vi "Thread@ForeachBreak__Parameter.vi"(1 "ParamterIn":string) -> (0 "ParamterOut":string)   [LabVIEW 2019]
panel:
  out "Variable List":string[](array[string])
  in  "Confirm":bool
  out "IO List":string[](array[string])
  in  "IOLogic":string(combo)
  # "Thread@ForeachBreak $IOLogic\nIOLogic Express is:\nIO1 & (IO2 | IO3)\nVar==XXX, !=XXX, >=XXX, <=XXX, >XXX, <XXX\nVar <> XXX~YYY, </>XXX~YYY\nVar==NULL, ==EXIST, ==[],==[;;]\n~IOLogic will inverse Logic"
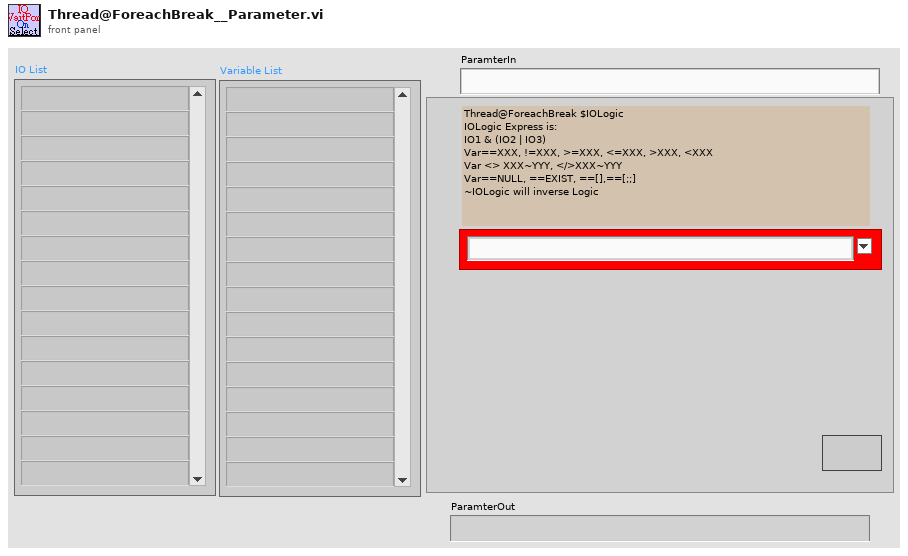
[diagram p1: front panel]
types:
  T1 = enum16{"Get", "Init", "Set", "Delete", "GetElement", "Inc", "Dec", "ReName"}
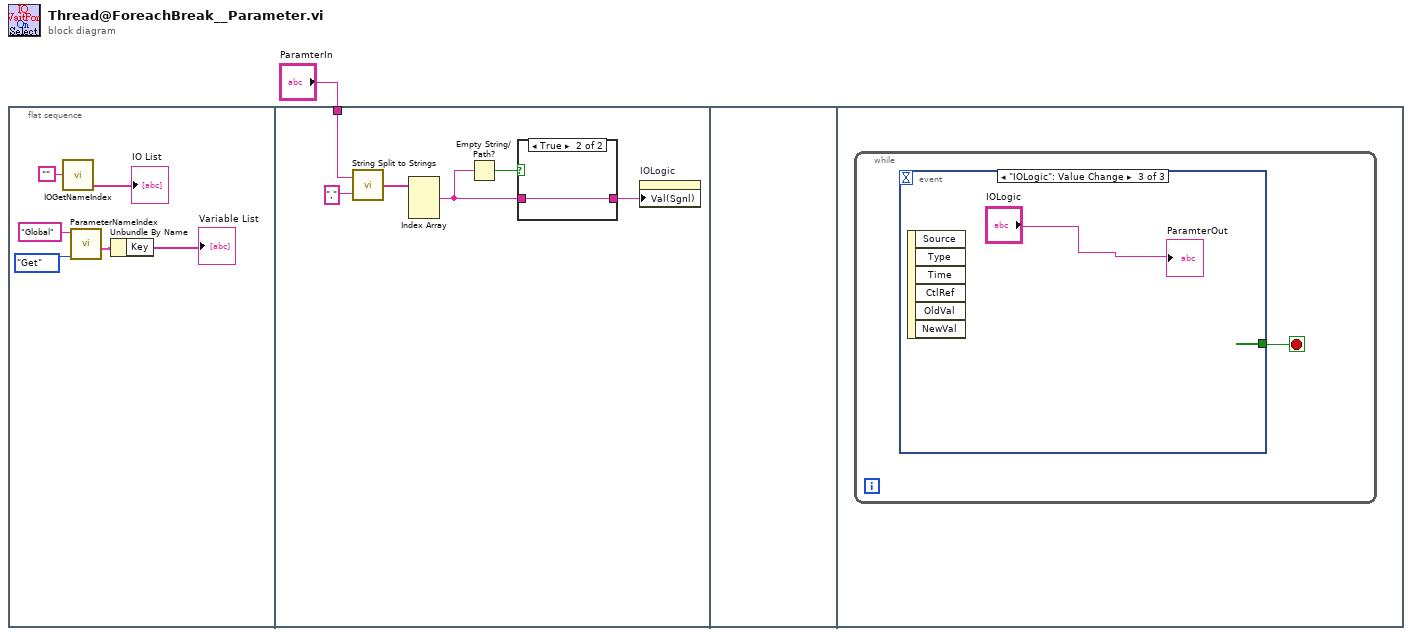
[diagram p0: block diagram]
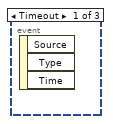
[diagram p3: hidden frame]
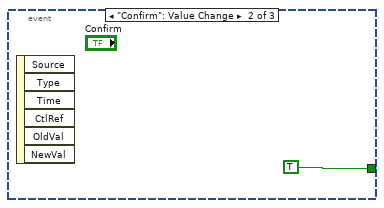
[diagram p4: hidden frame]
diagram:
  n1 = flat-sequence {
    tunnel: "ParamterIn" -> [w12]
    frame #0 {
      n2 = call "IOGetNameIndex.vi"("PortName"="") -> ("PortNameList Out"=→"IO List":string[])  [unwired: 3 in, 1 out]
      n3 = call "ParameterNameIndex.vi"("OP"=T1."Get", "VariableSection"="Global") -> ("GlobalKeyValue"=w4:cluster{"Key":string[], "Value":string[]})  [unwired: 3 in, 6 out]
      n4 = Unbundle By Name(w4) -> ("Key"=→"Variable List":string[])
    }
    frame #1 {
      n5 = call "String Split to Strings.vi"("search string/char (-)"=",", "String"=w12) -> ("Array"=w11:string[])
      n6 = Index Array(array=w11) -> (element #1=w9:string)  [unwired: 3 in, 2 out]
      n7 = Empty String/Path?(string/path=w9) -> (empty?=w10:bool)
      n8 = case shown="True" w10 {
        tunnel: w9 -> [w14 w15]
        tunnel: [w14 w15] -> w8
        frame False {
        }
        frame True {
        }
      }
      n9 = property on="IOLogic" class="CmbBox"("Val(Sgnl)"=w8) -> ()  [unwired: 2 in, 2 out]
    }
    frame #2 {
    }
    frame #3 {
      n10 = while {
        stop <- w16 stop-if-true
        n11 = event shown="[2] \"IOLogic\": Value Change" {
          selector: _ -> [_ _ _]
          dyn-events: _ -> [_ _ _]
          timeout: _ -> [_ _ _]
          tunnel: [_ TRUE _] -> w16
          event Timeout {
            n12 = event-data() -> ()  [unwired: 1 in, 3 out]
          }
          event "Confirm": Value Change {
            n13 = event-data() -> ()  [unwired: 1 in, 6 out]
          }
          event "IOLogic": Value Change {
            n14 = event-data() -> ()  [unwired: 1 in, 6 out]
            "ParamterOut" <- "IOLogic"
          }
        }
      }
    }
  }
